vi "Get interface status.vi"(8 "error in (no error)":errorcluster, 11 "RxTx in":refnum<class "RxTx.lvclass">) -> (0 "error out":errorcluster, 3 "RxTx out":refnum<class "RxTx.lvclass">)   [LabVIEW 2018, in "RxTx.lvclass"]
uses:
  RxTx.lvclass
  Interface/Interface.lvclass
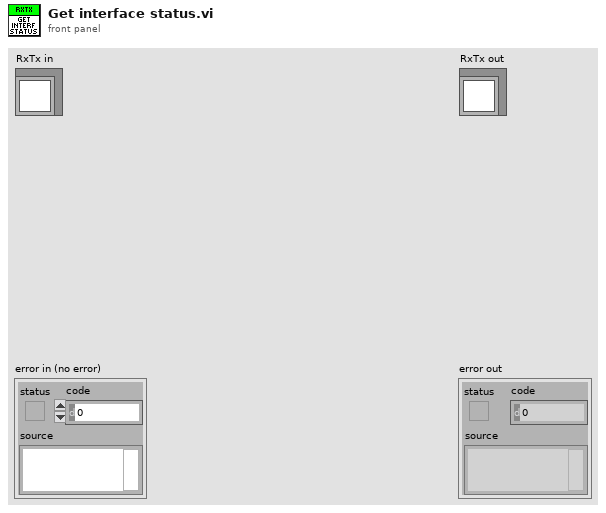
[diagram p1: front panel]
types:
  T1 = cluster{"Current Temperature":i16, "Temperatue Status":string}
  T2 = cluster{"Initialization":bool, "Serial Number":u16}
  T3 = cluster{"Exposure Time":sgl, "Pre-amp gain":u8, "Readout Rate":u8, "EM Mode":u8, "EM Gain":u16, "Binning":u16, "Initial Line":u16, "Initial Cloumn":u16, "Final Line":u16, "Final Column":u16, "Kinetic Series Length":u32, "Shutter Mode":u8, "Cooler ON/OFF":u16, "Temperature":i8, "Image Name":string, "Image Path":string, "#Images":u32, "Trigger":u16}
  T4 = cluster{"Cube exposure time":sgl, "Cubes done":u16, "Last image name":string, "Disk Space":u16, "Frames done":u16, "CCD status":string, "Current Temperature":i16, "Temperatue Status":string, "Frames exposure time":u16}
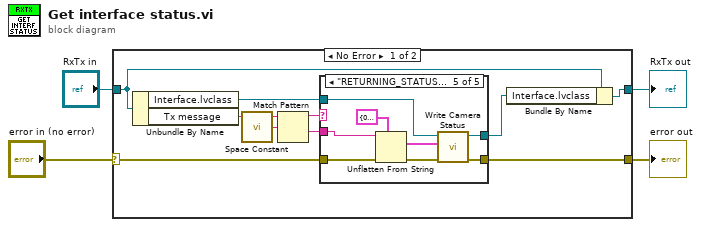
[diagram p0: block diagram]
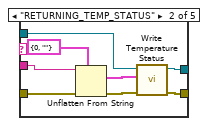
[diagram p3: hidden frame]
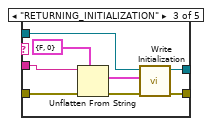
[diagram p4: hidden frame]
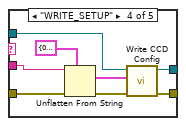
[diagram p5: hidden frame]
diagram:
  n1 = case shown="No Error" "error in (no error)" {
    selector: "error in (no error)" -> [w8 w50]
    tunnel: [w9 w50] -> w1
    tunnel: [w6 w49] -> w2
    tunnel: "RxTx in" -> [w7 w49]
    frame No Error {
      n2 = Unbundle By Name(w7) -> ("Interface.lvclass"=w11:refnum<class "Interface.lvclass">, "Tx message"=w10:string)
      n3 = call <vilib>:"Space Constant.vi"() -> ("String"=w14:string)
      n4 = Match Pattern(string=w10, regular expression=w14) -> (before substring=w5:string, after substring=w13:string)  [unwired: 1 in, 2 out]
      n5 = case shown="\"RETURNING_STATUS\"" w5 {
        tunnel: w13 -> [_ w24 w26 w35 w43]
        tunnel: [w16 w23 w29 w37 w45] -> w12
        tunnel: w11 -> [w16 w22 w30 w36 w44]
        tunnel: [w15 w18 w28 w38 w46] -> w9
        tunnel: w8 -> [w15 w17 w27 w39 w47]
        frame "False", Default {
        }
        frame "RETURNING_TEMP_STATUS" {
          n6 = Unflatten From String(type=T1 {"Current Temperature"=0, "Temperatue Status"=""} ("Temperature Status"), binary string=w24, error in (no error)=w17) -> (value=w20:T1, error out=w21:errorcluster)  [unwired: 2 in, 1 out]
          n7 = call "Write Temperature Status.vi"("error in (no error)"=w21, "Temperature Status"=w20, "Interface in"=w22) -> ("error out"=w18:errorcluster, "Interface out"=w23:refnum<class "Interface.lvclass">)  [unwired: 7 in]
        }
        frame "RETURNING_INITIALIZATION" {
          n8 = Unflatten From String(type=T2 {"Initialization"=FALSE, "Serial Number"=0} ("Initialization"), binary string=w26, error in (no error)=w27) -> (value=w25:T2, error out=w32:errorcluster)  [unwired: 2 in, 1 out]
          n9 = call "Write Initialization.vi"("error in (no error)"=w32, "Initialization"=w25, "Interface in"=w30) -> ("error out"=w28:errorcluster, "Interface out"=w29:refnum<class "Interface.lvclass">)  [unwired: 7 in]
        }
        frame "WRITE_SETUP" {
          n10 = Unflatten From String(type=T3 {"Exposure Time"=0.0, "Pre-amp gain"=0, "Readout Rate"=0, "EM Mode"=0, "EM Gain"=0, "Binning"=0, "Initial Line"=0, "Initial Cloumn"=0, "Final Line"=0, "Final Column"=0, "Kinetic Series Length"=0, "Shutter Mode"=0, "Cooler ON/OFF"=0, "Temperature"=0, "Image Name"="", "Image Path"="", "#Images"=0, "Trigger"=0} ("CCD Config"), binary string=w35, error in (no error)=w39) -> (value=w34:T3, error out=w40:errorcluster)  [unwired: 2 in, 1 out]
          n11 = call "Write CCD Config.vi"("error in (no error)"=w40, "CCD Config"=w34, "Interface in"=w36) -> ("error out"=w38:errorcluster, "Interface out"=w37:refnum<class "Interface.lvclass">)  [unwired: 7 in]
        }
        frame "RETURNING_STATUS" {
          n12 = Unflatten From String(type=T4 {"Cube exposure time"=0.0, "Cubes done"=0, "Last image name"="", "Disk Space"=0, "Frames done"=0, "CCD status"="", "Current Temperature"=0, "Temperatue Status"="", "Frames exposure time"=0} ("Camera Status"), binary string=w43, error in (no error)=w47) -> (value=w42:T4, error out=w48:errorcluster)  [unwired: 2 in, 1 out]
          n13 = call "Write Camera Status.vi"("error in (no error)"=w48, "Camera Status"=w42, "Interface in"=w44) -> ("error out"=w46:errorcluster, "Interface out"=w45:refnum<class "Interface.lvclass">)  [unwired: 7 in]
        }
      }
      n14 = Bundle By Name(cluster=w7, "Interface.lvclass"=w12) -> (w6:refnum<class "RxTx.lvclass">)
    }
    frame Error {
    }
  }
  "error out" <- w1
  "RxTx out" <- w2
